vi "Translate.vi"(10 "Message In":refnum<class "MSG.lvclass">, 11 "Translator in":refnum<class "Relabel.lvclass">) -> (2 "Translated Message":refnum<class "MSG.lvclass">, 3 "Translator out":refnum<class "Relabel.lvclass">)   [LabVIEW 2011, in "Messenging.lvlib" / "Relabel.lvclass"]
uses:
  Relabel.lvclass
  TextVarientMessage/MSG.lvclass
  Relabel.lvclass/Relabel.ctl
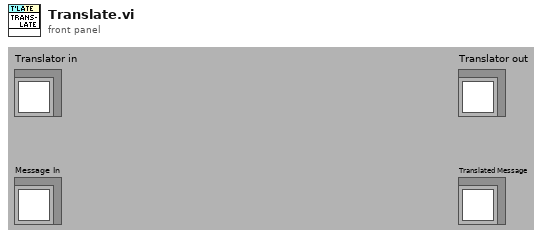
[diagram p1: front panel]
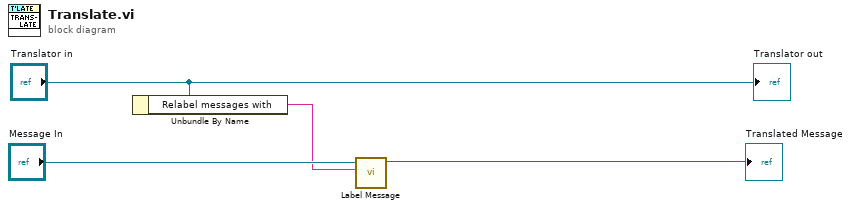
[diagram p0: block diagram]
diagram:
  n1 = Unbundle By Name("Translator in") -> ("Relabel messages with"=w1:string)
  n2 = call-dynamic "Label Message.vi"("Label"=w1, "Message"="Message In") -> ("Message"=→"Translated Message":refnum<class "MSG.lvclass">)  [unwired: 1 in, 8 out]
  "Translator out" <- "Translator in"
